vi "Get DOF Limits.vi"(10 "ID":T2, 11 "DofType":T1) -> (1 "Limits 3":cluster{"Lower":dbl, "Upper":dbl, "Actual":dbl}, 2 "Limits  4":cluster{"Lower":dbl, "Upper":dbl, "Actual":dbl}, 3 "Limits 5":cluster{"Lower":dbl, "Upper":dbl, "Actual":dbl}, 4 "Limits 2":cluster{"Lower":dbl, "Upper":dbl, "Actual":dbl}, 5 "Limits 6":cluster{"Lower":dbl, "Upper":dbl, "Actual":dbl}, 6 "Limits 1":cluster{"Lower":dbl, "Upper":dbl, "Actual":dbl})   [LabVIEW 2013]
uses:
  Data Access Objects/Metadata/LBCB Number.ctl
  Data Access Objects/Limits/DofTypes.ctl
  Data Access Objects/Metadata/Persistant DAO Actions.ctl
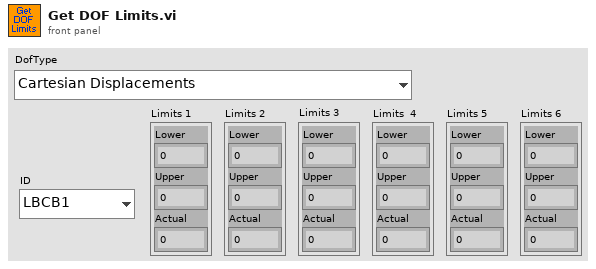
[diagram p1: front panel]
types:
  T1 = typedef "DofTypes.ctl" = enum16{"Cartesian Displacements", "Cartesian Forces & Moments", "Actuator Displacements", "Actuator Forces", "Cartesian Increments", "Actuator Increments"}
  T2 = typedef "LBCB Number.ctl" = enum16{"LBCB1", "LBCB2"}
  T3 = typedef "Persistant DAO Actions.ctl" = enum16{"Init", "Get", "Set", "Load", "Save"}
  T4 = typedef "Cartesian Matrix.ctl" = cluster{"Lower":T5, "Upper":T5}
  T5 = typedef "Cartesian Point.ctl" = cluster{"Dx":dbl, "Dy":dbl, "Dz":dbl, "Rx":dbl, "Ry":dbl, "Rz":dbl}
  T6 = typedef "Actuator Point.ctl" = cluster{"X1":dbl, "X2":dbl, "Y1":dbl, "Z1":dbl, "Z2":dbl, "Z3":dbl}
  T7 = typedef "Actuator Matrix.ctl" = cluster{"Lower":T6, "Upper":T6}
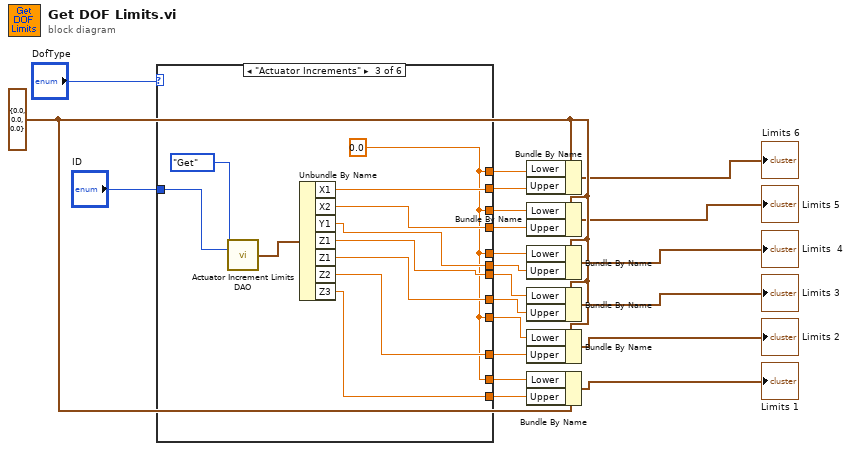
[diagram p0: block diagram]
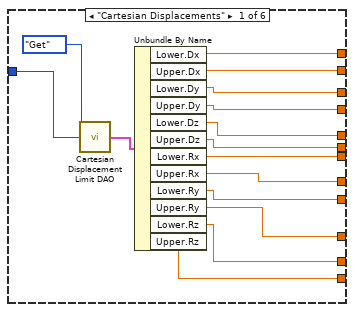
[diagram p2: hidden frame]
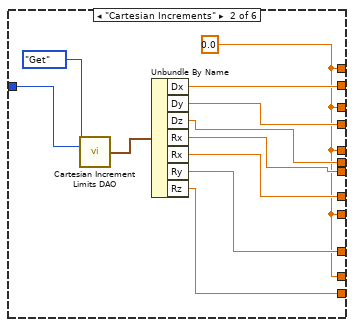
[diagram p3: hidden frame]
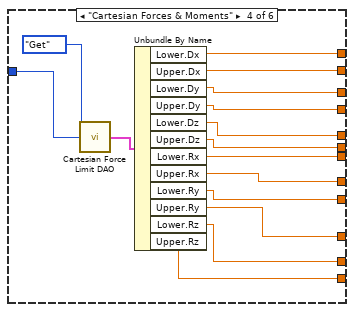
[diagram p4: hidden frame]
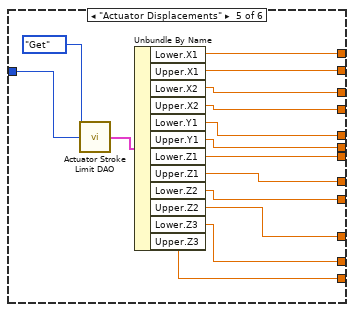
[diagram p5: hidden frame]
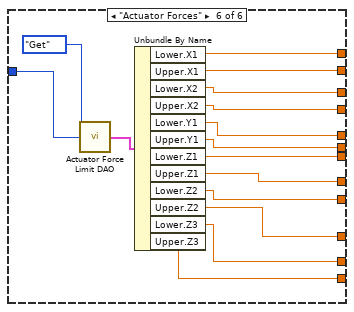
[diagram p6: hidden frame]
diagram:
  w17 = cluster{"Lower":dbl, "Upper":dbl, "Actual":dbl} {"Lower"=0.0, "Upper"=0.0, "Actual"=0.0} ("Limits X 5")
  n1 = case shown="\"Actuator Increments\"" "DofType" {
    tunnel: [w36 w47 w58 w73 w88 w103] -> w15
    tunnel: [w35 w37 w48 w72 w87 w102] -> w14
    tunnel: [w34 w46 w57 w71 w86 w101] -> w13
    tunnel: [w33 w37 w48 w70 w85 w100] -> w12
    tunnel: [w32 w45 w56 w69 w84 w99] -> w11
    tunnel: [w31 w44 w55 w68 w83 w98] -> w10
    tunnel: [w30 w43 w54 w67 w82 w97] -> w9
    tunnel: [w29 w37 w48 w66 w81 w96] -> w8
    tunnel: [w28 w42 w53 w65 w80 w95] -> w7
    tunnel: [w27 w37 w48 w64 w79 w94] -> w6
    tunnel: [w26 w41 w52 w63 w78 w93] -> w4
    tunnel: [w25 w37 w48 w62 w77 w92] -> w3
    tunnel: "ID" -> [w22 w38 w49 w59 w74 w89]
    frame "Cartesian Displacements" {
      n2 = call "Cartesian Displacement Limit DAO.vi"("Cartesian Displacement Limit Actions"=Persistant_DAO_Actions."Get", "ID"=w22) -> ("Cartesian Displacement Out"=w24:T4)  [unwired: 11 in, 2 out]
      n3 = Unbundle By Name(w24) -> ("Lower.Dx"=w25:dbl, "Upper.Dx"=w26:dbl, "Lower.Dy"=w27:dbl, "Upper.Dy"=w28:dbl, "Lower.Dz"=w29:dbl, "Upper.Dz"=w30:dbl, "Lower.Rx"=w31:dbl, "Upper.Rx"=w32:dbl, "Lower.Ry"=w33:dbl, "Upper.Ry"=w34:dbl, "Lower.Rz"=w35:dbl, "Upper.Rz"=w36:dbl)
    }
    frame "Cartesian Increments" {
      w37 = 0.0 ("X1")
      n4 = call "Cartesian Increment Limits DAO.vi"("Actions"=Persistant_DAO_Actions."Get" ("Cartesian Displacement Limit Actions"), "LBCB Number"=w38) -> ("Inc Limits Out"=w40:T5)  [unwired: 11 in, 2 out]
      n5 = Unbundle By Name(w40) -> ("Dx"=w41:dbl, "Dy"=w42:dbl, "Dz"=w43:dbl, "Rx"=w44:dbl, "Rx"=w45:dbl, "Ry"=w46:dbl, "Rz"=w47:dbl)
    }
    frame "Actuator Increments" {
      w48 = 0.0 ("X1")
      n6 = call "Actuator Increment Limits DAO.vi"("Actions"=Persistant_DAO_Actions."Get" ("Cartesian Displacement Limit Actions"), "LBCB Number"=w49) -> ("Inc Limits Out"=w51:T6)  [unwired: 11 in, 2 out]
      n7 = Unbundle By Name(w51) -> ("X1"=w52:dbl, "X2"=w53:dbl, "Y1"=w54:dbl, "Z1"=w55:dbl, "Z1"=w56:dbl, "Z2"=w57:dbl, "Z3"=w58:dbl)
    }
    frame "Cartesian Forces & Moments" {
      n8 = call "Cartesian Force Limit DAO.vi"("Cartesian Force Limit Actions"=Persistant_DAO_Actions."Get" ("Cartesian Displacement Limit Actions"), "ID"=w59) -> ("Cartesian Force Limit Out"=w61:T4)  [unwired: 11 in, 2 out]
      n9 = Unbundle By Name(w61) -> ("Lower.Dx"=w62:dbl, "Upper.Dx"=w63:dbl, "Lower.Dy"=w64:dbl, "Upper.Dy"=w65:dbl, "Lower.Dz"=w66:dbl, "Upper.Dz"=w67:dbl, "Lower.Rx"=w68:dbl, "Upper.Rx"=w69:dbl, "Lower.Ry"=w70:dbl, "Upper.Ry"=w71:dbl, "Lower.Rz"=w72:dbl, "Upper.Rz"=w73:dbl)
    }
    frame "Actuator Displacements" {
      n10 = call "Actuator Stroke Limit DAO.vi"("Actuator Stroke Limit Actions"=Persistant_DAO_Actions."Get" ("Cartesian Displacement Limit Actions"), "ID"=w74) -> ("Actuator Stroke Limits Out"=w76:T7)  [unwired: 11 in, 2 out]
      n11 = Unbundle By Name(w76) -> ("Lower.X1"=w77:dbl, "Upper.X1"=w78:dbl, "Lower.X2"=w79:dbl, "Upper.X2"=w80:dbl, "Lower.Y1"=w81:dbl, "Upper.Y1"=w82:dbl, "Lower.Z1"=w83:dbl, "Upper.Z1"=w84:dbl, "Lower.Z2"=w85:dbl, "Upper.Z2"=w86:dbl, "Lower.Z3"=w87:dbl, "Upper.Z3"=w88:dbl)
    }
    frame "Actuator Forces" {
      n12 = call "Actuator Force Limit DAO.vi"("Actuator Force Limit Actions"=Persistant_DAO_Actions."Get" ("Cartesian Displacement Limit Actions"), "ID"=w89) -> ("Actuator Force Limits Out"=w91:T7)  [unwired: 11 in, 2 out]
      n13 = Unbundle By Name(w91) -> ("Lower.X1"=w92:dbl, "Upper.X1"=w93:dbl, "Lower.X2"=w94:dbl, "Upper.X2"=w95:dbl, "Lower.Y1"=w96:dbl, "Upper.Y1"=w97:dbl, "Lower.Z1"=w98:dbl, "Upper.Z1"=w99:dbl, "Lower.Z2"=w100:dbl, "Upper.Z2"=w101:dbl, "Lower.Z3"=w102:dbl, "Upper.Z3"=w103:dbl)
    }
  }
  n14 = Bundle By Name(cluster=w17, "Lower"=w3, "Upper"=w4) -> (→"Limits 6":cluster{"Lower":dbl, "Upper":dbl, "Actual":dbl})
  n15 = Bundle By Name(cluster=w17, "Lower"=w6, "Upper"=w7) -> (→"Limits 5":cluster{"Lower":dbl, "Upper":dbl, "Actual":dbl})
  n16 = Bundle By Name(cluster=w17, "Lower"=w8, "Upper"=w9) -> (→"Limits  4":cluster{"Lower":dbl, "Upper":dbl, "Actual":dbl})
  n17 = Bundle By Name(cluster=w17, "Lower"=w10, "Upper"=w11) -> (→"Limits 3":cluster{"Lower":dbl, "Upper":dbl, "Actual":dbl})
  n18 = Bundle By Name(cluster=w17, "Lower"=w12, "Upper"=w13) -> (→"Limits 2":cluster{"Lower":dbl, "Upper":dbl, "Actual":dbl})
  n19 = Bundle By Name(cluster=w17, "Lower"=w14, "Upper"=w15) -> (→"Limits 1":cluster{"Lower":dbl, "Upper":dbl, "Actual":dbl})
